vi "HT_Locate_allocate.vi"(8 "error in (no error)":errorcluster, 11 "session in":refnum<k35>) -> (0 "error out":errorcluster, 2 "return value":string, 3 "Refnum out":refnum<k35>)   [LabVIEW 2023, in "holoTracker.lvlib"]
uses:
  holoTracker.lvlib
panel:
  # "wavelenght, optical_index, image_size_X, image_size_Y, pixel_size, magnification = holo_info\n\n    propag_param, focus_param, binarisation_param, CCL_param = analyse_parameters\n    distance_ini, nb_plane, propag_step, filter = propag_param\n    high_pass_filter, low_pass_filter = filter\n    #focus parameters unpacking\n    focus_type, sum_size = focus_param\n    #binarisation parameters unpacking\n    nbStdVarThreshold, threshold_target = binarisation_param\n    #CCL parameters unpacking\n    n_connectivity, min_voxel, max_voxel = CCL_param"
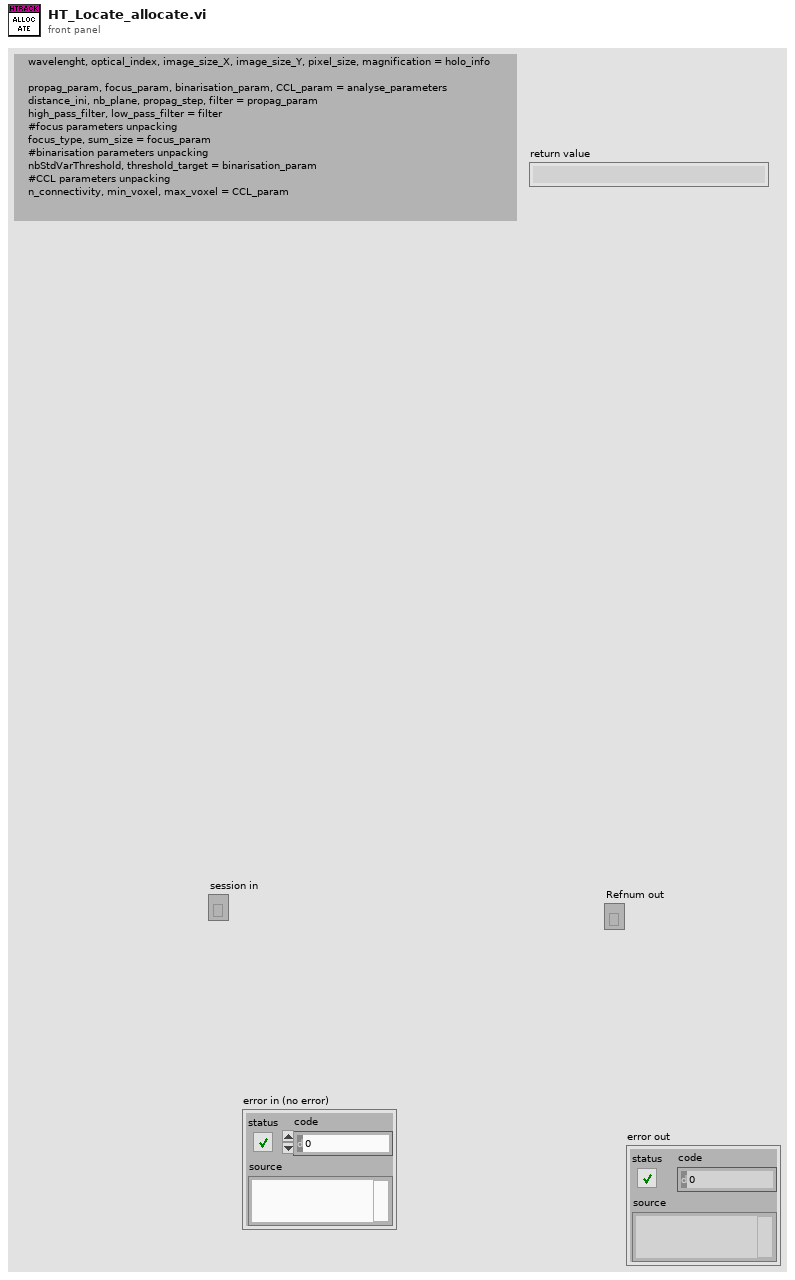
[diagram p1: front panel]
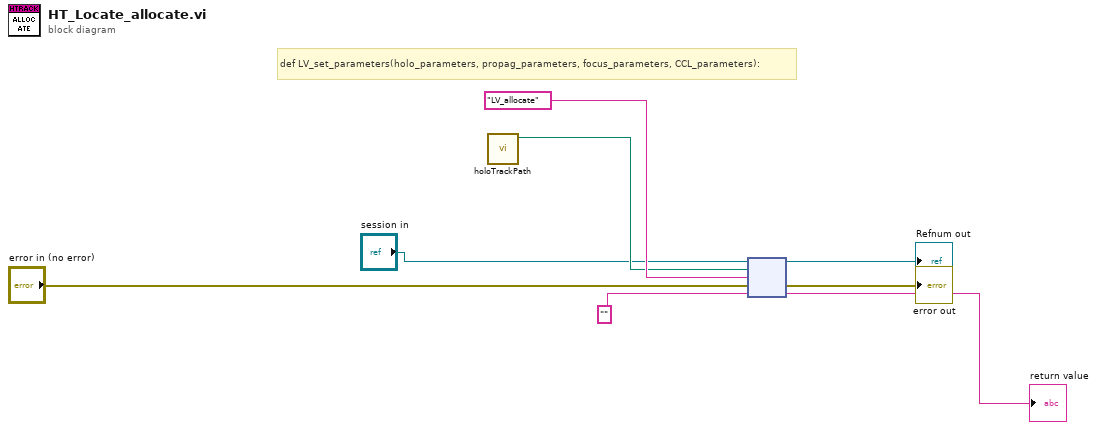
[diagram p0: block diagram]
diagram:
  # "def LV_set_parameters(holo_parameters, propag_parameters, focus_parameters, CCL_parameters):"
  n1 = call "holoTrackPath.vi"() -> ("appended path"=w3:path)  [unwired: 11 in]
  n2 = node("session in", w3, "LV_allocate" ("function name"), "error in (no error)", "") -> (→"Refnum out":refnum<k35>, →"error out":errorcluster, →"return value":string)  [unwired: 2 out]
